vi "MSScript_Exe_Command.vi"(8 "error in (no error)":errorcluster, 9 "Expression index":i32, 11 "MSScript in":refnum<class "MSScript.lvclass">) -> (0 "Error out":errorcluster, 1 "Next expression index":i32, 3 "MSScript out":refnum<class "MSScript.lvclass">)   [LabVIEW 2018, in "MSScript.lvclass"]
uses:
  MSScript.lvclass
  MSScript.lvclass/MSScript.ctl
  MSScript_Error_(6008)UnknownCmd.vi
  MSScript_Error_(6007)CalcError.vi
  MSScript_Error_(6006)ParamErr.vi
  MSScript_Error_(6010)CommentLost.vi
  MSScript_Error_(6000)VariableNoFound.vi
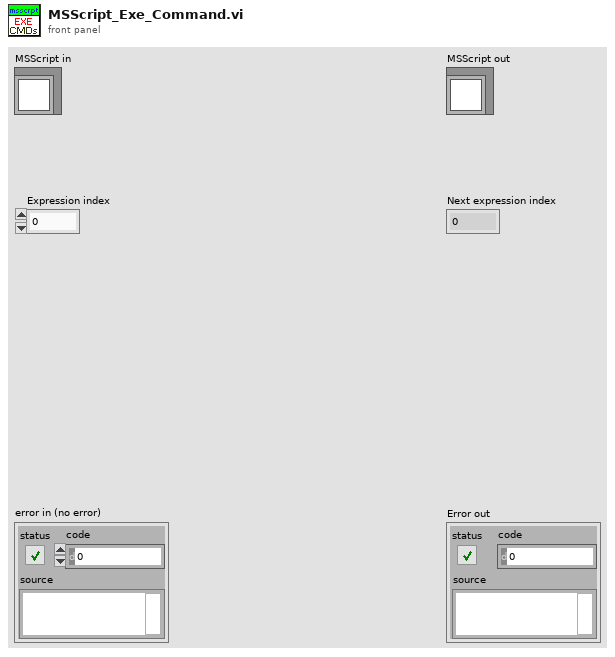
[diagram p1: front panel]
types:
  T1 = cluster{"Type":string, "NAME":cluster{"STR":string, "Start":i32}, "PARAMs":cluster{"STR":string, "Start":i32}[]}[]
  T2 = cluster{"Type":string, "NAME":cluster{"STR":string, "Start":i32}, "PARAMs":cluster{"STR":string, "Start":i32}[]}
  T3 = enum16{"Scalar", "ScalarArray", "Var", "VarArray", "Error"}
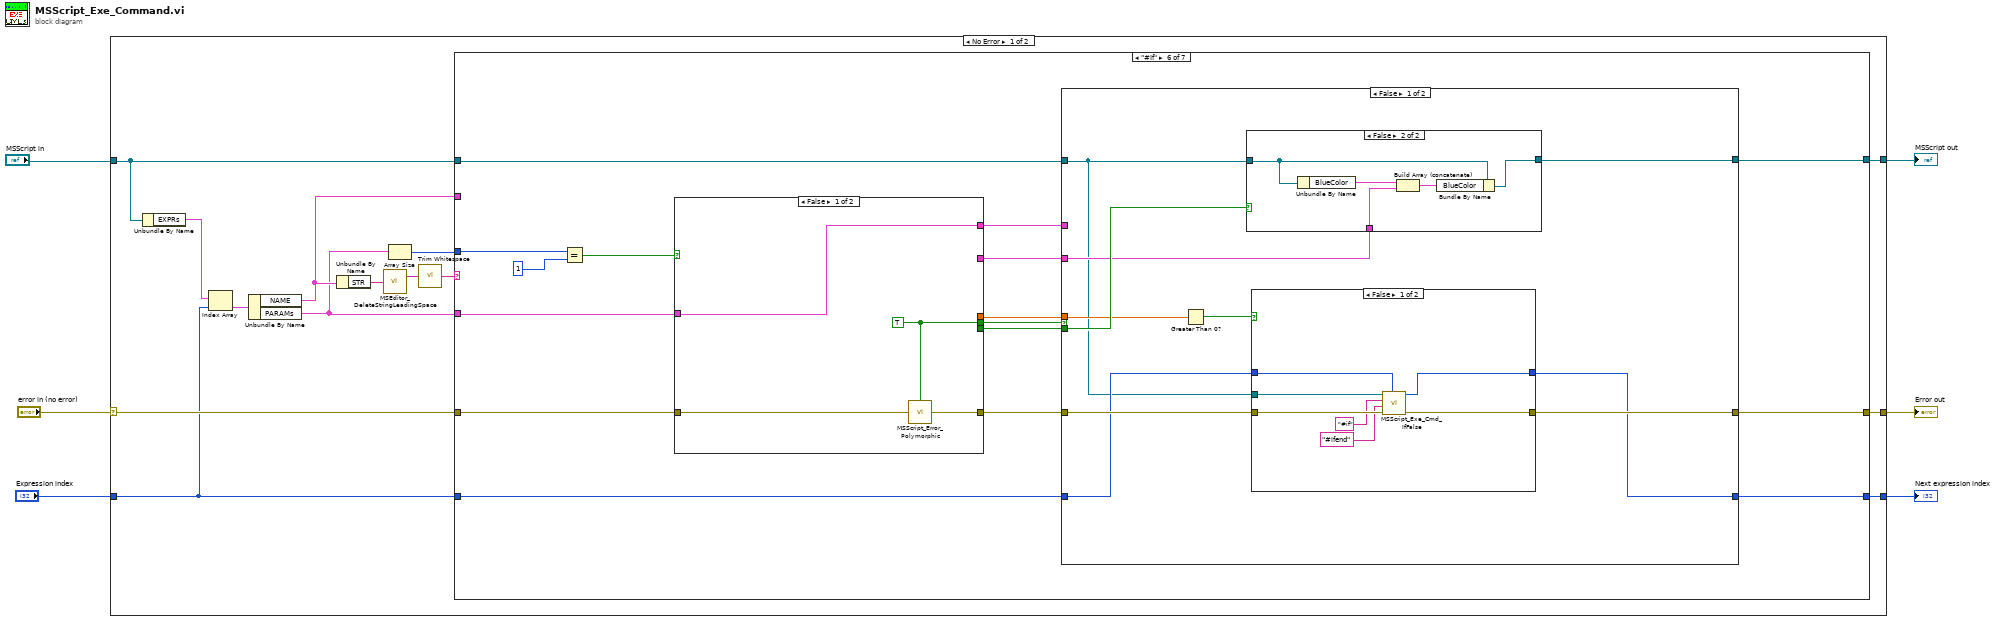
[diagram p0: block diagram]
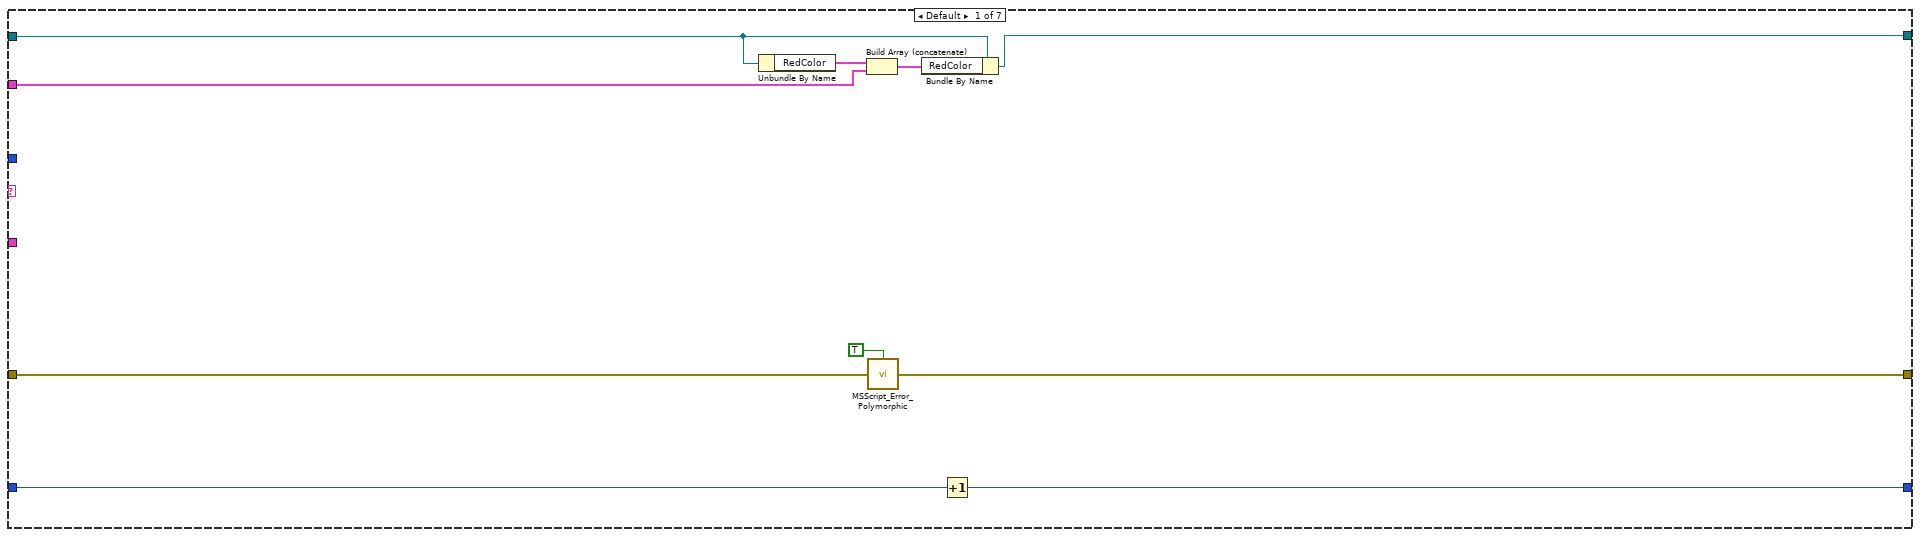
[diagram p2: hidden frame]
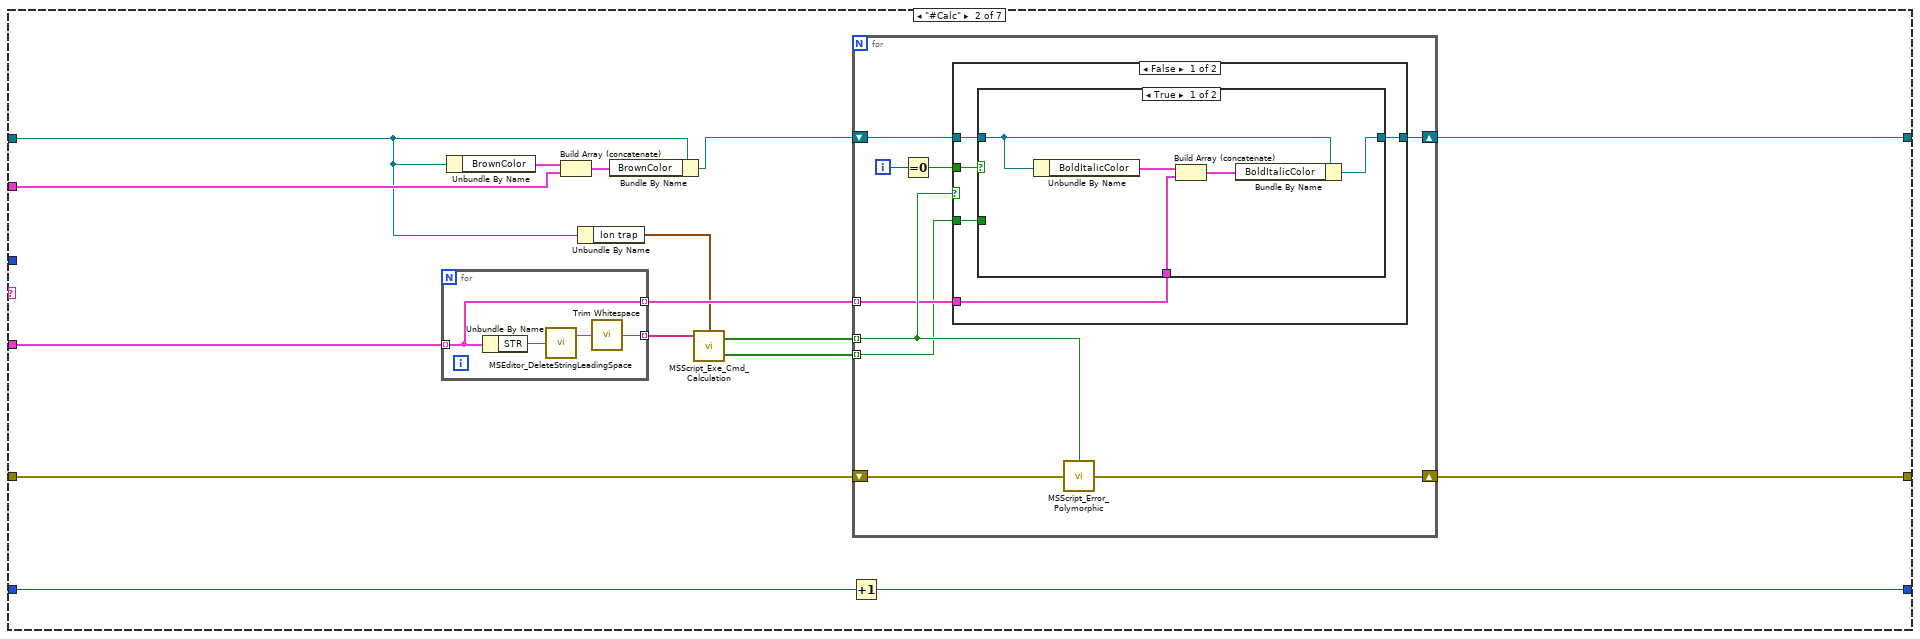
[diagram p3: hidden frame]
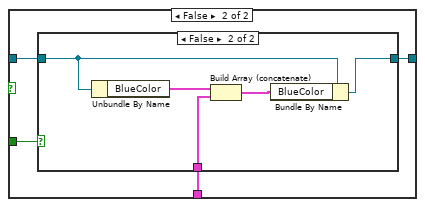
[diagram p4: hidden frame]
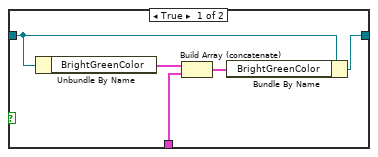
[diagram p5: hidden frame]
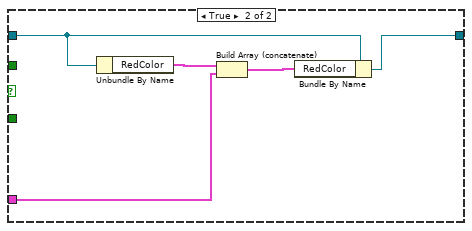
[diagram p6: hidden frame]
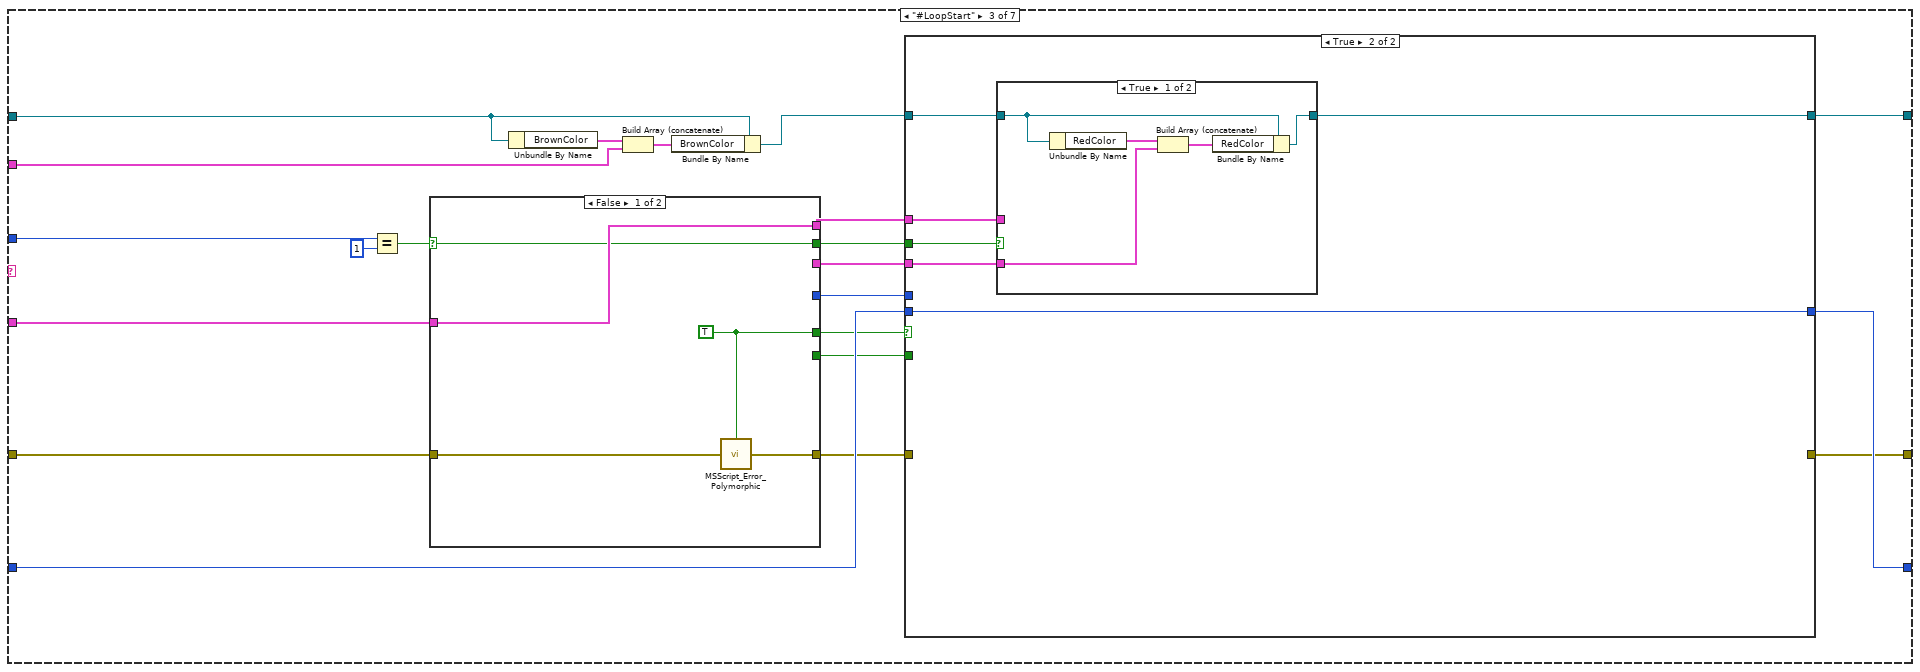
[diagram p7: hidden frame]
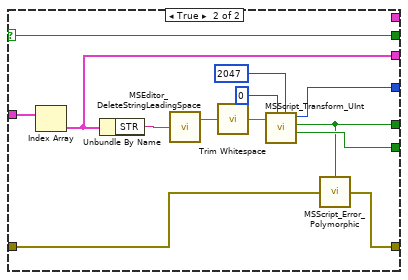
[diagram p8: hidden frame]
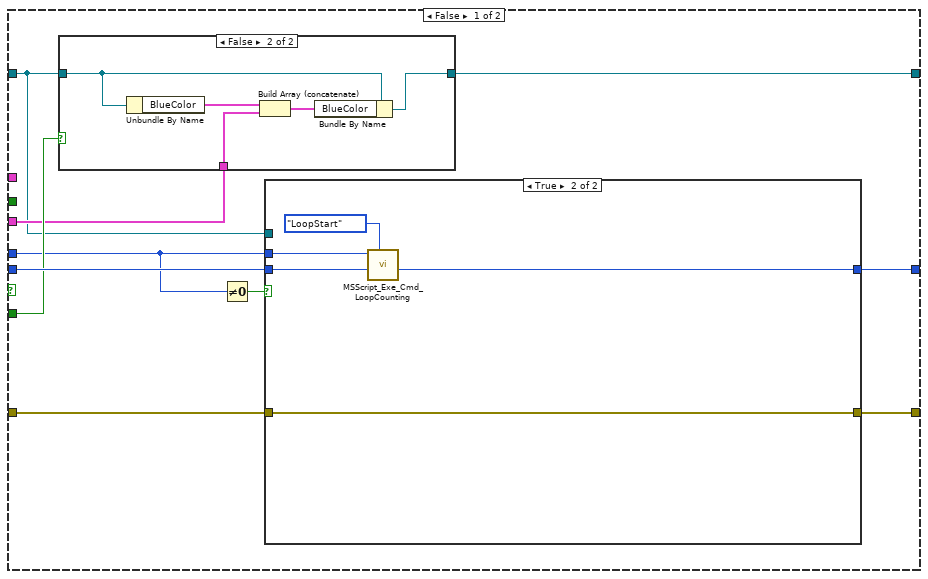
[diagram p9: hidden frame]
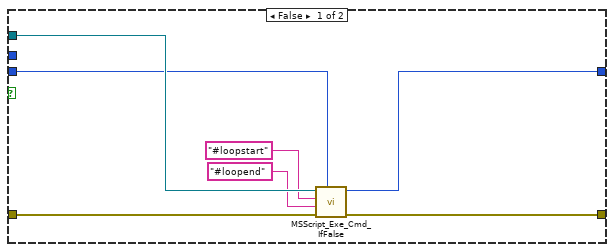
[diagram p10: hidden frame]
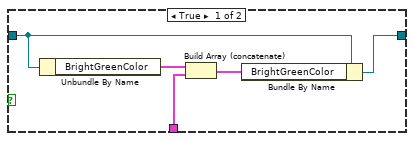
[diagram p11: hidden frame]
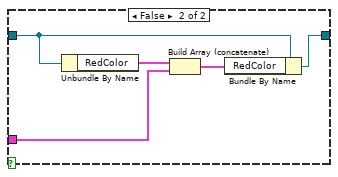
[diagram p12: hidden frame]
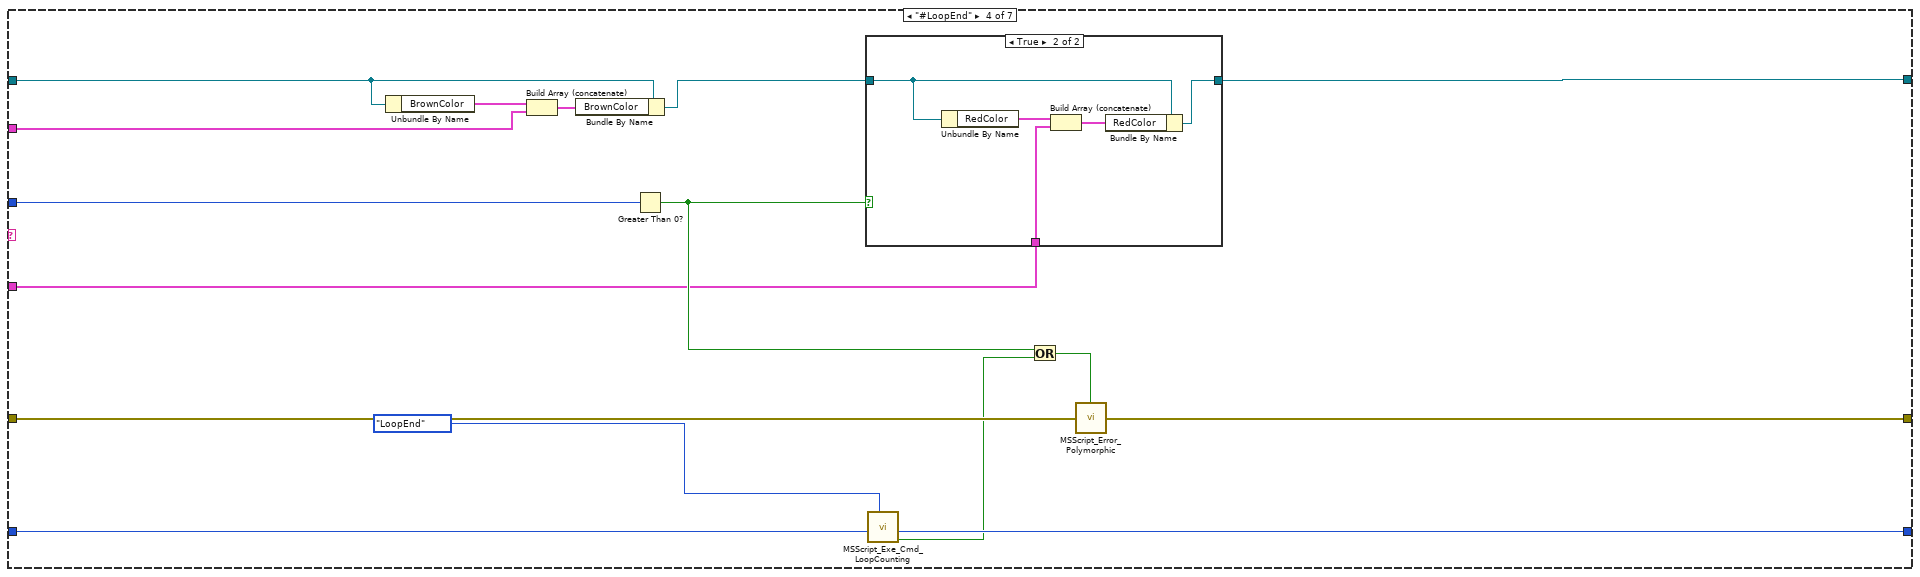
[diagram p13: hidden frame]
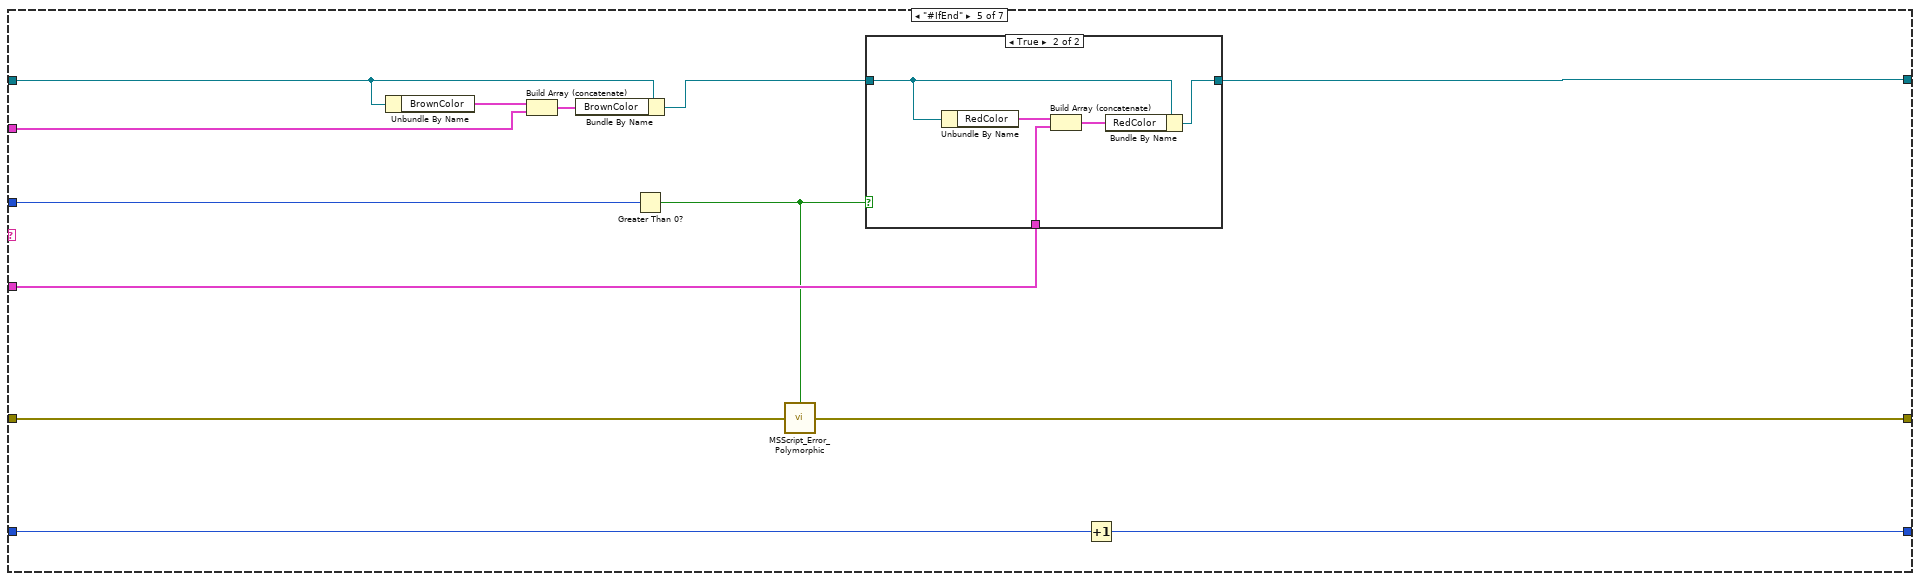
[diagram p15: hidden frame]
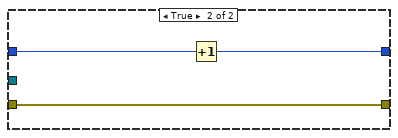
[diagram p17: hidden frame]
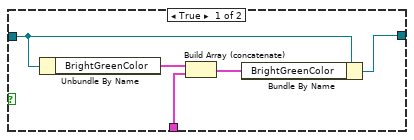
[diagram p18: hidden frame]
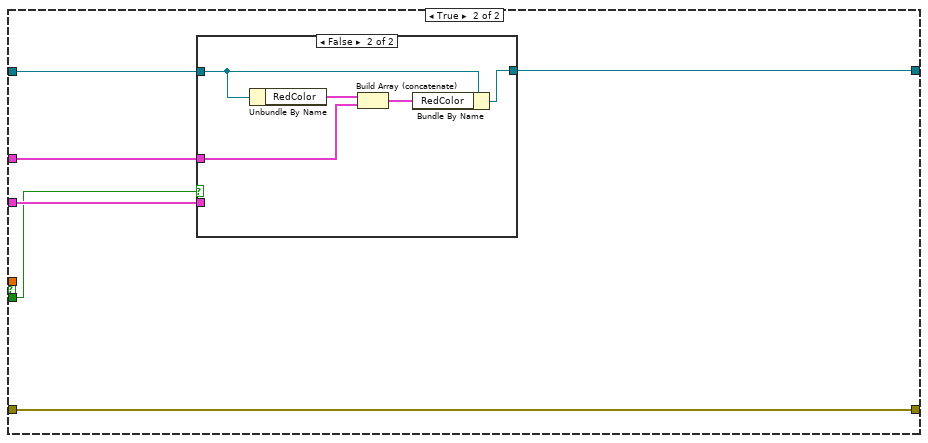
[diagram p19: hidden frame]
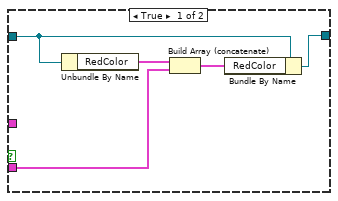
[diagram p20: hidden frame]
diagram:
  n1 = case shown="No Error" "error in (no error)" {
    selector: "error in (no error)" -> [w17 w388]
    tunnel: [w20 w386] -> w6
    tunnel: "MSScript in" -> [w7 w385]
    tunnel: "Expression index" -> [w8 w387]
    tunnel: [w16 w388] -> w2
    tunnel: [w12 w385] -> w1
    frame No Error {
      n2 = Unbundle By Name(w7) -> ("EXPRs"=w19:T1)
      n3 = Index Array(array=w19, index=w8) -> (element=w18:T2)
      n4 = Unbundle By Name(w18) -> ("NAME"=w11:cluster{"STR":string, "Start":i32}, "PARAMs"=w10:cluster{"STR":string, "Start":i32}[])
      n5 = Unbundle By Name(w11) -> ("STR"=w15:string)
      n6 = call "MSEditor_DeleteStringLeadingSpace.vi"("string in"=w15) -> ("string after leading space"=w14:string)  [unwired: 1 out]
      n7 = Array Size(array=w10) -> (size(s)=w9:i32)
      n8 = call <vilib>:"Trim Whitespace.vi"("string"=w14) -> ("trimmed string"=w13:string)  [unwired: 1 in]
      n9 = case shown="\"#If\"" w13 {
        tunnel: w10 -> [_ w44 w109 w176 w201 w228 w312]
        tunnel: w8 -> [w29 w45 w108 w190 w200 w218 w316]
        tunnel: [w30 w46 w107 w189 w199 w217 w317] -> w20
        tunnel: w17 -> [w28 w43 w106 w188 w210 w232 w305]
        tunnel: [w27 w42 w89 w187 w209 w221 w296] -> w16
        tunnel: w11 -> [w23 w36 w104 w185 w207 _ w315]
        tunnel: w7 -> [w22 w32 w105 w186 w208 w224 w314]
        tunnel: [w21 w34 w103 w177 w202 w220 w313] -> w12
        tunnel: w9 -> [_ _ w102 w184 w206 w230 w311]
        frame Default {
          n10 = Unbundle By Name(w22) -> ("RedColor"=w25:cluster{"STR":string, "Start":i32}[])
          n11 = Build Array (concatenate)(w25, w23) -> (w24:cluster{"STR":string, "Start":i32}[])
          n12 = call-poly "MSScript_Error_Polymorphic.vi"("error in (no error)"=w28, "ErrBoolean"=TRUE) -> ("error out"=w27:errorcluster)
          n13 = Bundle By Name(cluster=w22, "RedColor"=w24) -> (w21:refnum<class "MSScript.lvclass">)
          n14 = Increment(x=w29) -> (x+1=w30:i32)
        }
        frame "#Calc" {
          n15 = for {
            tunnel: w44 -> [w85] mode=indexing
            tunnel: [w86] -> w41 mode=indexing
            tunnel: [w85] -> w39 mode=indexing
            n16 = Unbundle By Name(w85) -> ("STR"=w87:string)
            n17 = call "MSEditor_DeleteStringLeadingSpace.vi"("string in"=w87) -> ("string after leading space"=w88:string)  [unwired: 1 out]
            n18 = call <vilib>:"Trim Whitespace.vi"("string"=w88) -> ("trimmed string"=w86:string)  [unwired: 1 in]
          }
          n19 = Unbundle By Name(w32) -> ("BrownColor"=w38:cluster{"STR":string, "Start":i32}[])
          n20 = Build Array (concatenate)(w38, w36) -> (w37:cluster{"STR":string, "Start":i32}[])
          n21 = Unbundle By Name(w32) -> ("Ion trap"=w31:cluster{"R0":ext, "Z0":ext})
          n22 = Bundle By Name(cluster=w32, "BrownColor"=w37) -> (w35:refnum<class "MSScript.lvclass">)
          n23 = call "MSScript_Exe_Cmd_Calculation.vi"("Ion trap"=w31, "ValueArray"=w41) -> ("Is a variable?"=w33:bool[], "ErrorBooleanArray"=w40:bool[])  [unwired: 2 in]
          n24 = Increment(x=w45) -> (x+1=w46:i32)
          n25 = for {
            tunnel: w40 -> [w51] mode=indexing
            shift-right: [w54] -> w42
            shift-left: w43 -> [w55]
            tunnel: w39 -> [w50] mode=indexing
            tunnel: w33 -> [w49] mode=indexing
            shift-right: [w53] -> w34
            shift-left: w35 -> [w52]
            i -> [w48]
            n26 = Equal To 0?(x=w48) -> (x = 0?=w47:bool)
            n27 = case shown="False" w51 {
              tunnel: [w59 w83] -> w53
              tunnel: w52 -> [w60 w84]
              tunnel: w50 -> [w58 w81]
              tunnel: w49 -> [w57 _]
              tunnel: w47 -> [w56 _]
              frame False {
                n28 = case shown="True" w56 {
                  tunnel: w60 -> [w63 w69]
                  tunnel: [w62 w68] -> w59
                  tunnel: w58 -> [w61 w67]
                  tunnel: w57 -> [_ w66]
                  frame True {
                    n29 = Unbundle By Name(w63) -> ("BoldItalicColor"=w65:cluster{"STR":string, "Start":i32}[])
                    n30 = Build Array (concatenate)(w65, w61) -> (w64:cluster{"STR":string, "Start":i32}[])
                    n31 = Bundle By Name(cluster=w63, "BoldItalicColor"=w64) -> (w62:refnum<class "MSScript.lvclass">)
                  }
                  frame False {
                    n32 = case shown="False" w66 {
                      tunnel: w69 -> [w74 w79]
                      tunnel: [w73 w78] -> w68
                      tunnel: w67 -> [w71 w76]
                      frame True {
                        n33 = Unbundle By Name(w74) -> ("BrightGreenColor"=w72:cluster{"STR":string, "Start":i32}[])
                        n34 = Build Array (concatenate)(w72, w71) -> (w70:cluster{"STR":string, "Start":i32}[])
                        n35 = Bundle By Name(cluster=w74, "BrightGreenColor"=w70) -> (w73:refnum<class "MSScript.lvclass">)
                      }
                      frame False {
                        n36 = Unbundle By Name(w79) -> ("BlueColor"=w77:cluster{"STR":string, "Start":i32}[])
                        n37 = Build Array (concatenate)(w77, w76) -> (w75:cluster{"STR":string, "Start":i32}[])
                        n38 = Bundle By Name(cluster=w79, "BlueColor"=w75) -> (w78:refnum<class "MSScript.lvclass">)
                      }
                    }
                  }
                }
              }
              frame True {
                n39 = Unbundle By Name(w84) -> ("RedColor"=w82:cluster{"STR":string, "Start":i32}[])
                n40 = Build Array (concatenate)(w82, w81) -> (w80:cluster{"STR":string, "Start":i32}[])
                n41 = Bundle By Name(cluster=w84, "RedColor"=w80) -> (w83:refnum<class "MSScript.lvclass">)
              }
            }
            n42 = call-poly "MSScript_Error_Polymorphic.vi"("error in (no error)"=w55, "ErrBoolean"=w51) -> ("error out"=w54:errorcluster)
          }
        }
        frame "#LoopStart" {
          n43 = Equal?(x=w102, y=1) -> (x = y?=w100:bool)
          n44 = case shown="False" w100 {
            selector: w100 -> [w113 w118]
            tunnel: w109 -> [w114 w127]
            tunnel: [_ w124] -> w99
            tunnel: [_ w120] -> w98
            tunnel: [w110 w115] -> w95
            tunnel: [_ w119] -> w93
            tunnel: [w114 _] -> w92
            tunnel: [w113 w118] -> w91
            tunnel: w106 -> [w112 w117]
            tunnel: [w111 w116] -> w90
            frame False {
              w110 = TRUE
              n45 = call-poly "MSScript_Error_Polymorphic.vi"("error in (no error)"=w112, "ErrBoolean"=w110) -> ("error out"=w111:errorcluster)
            }
            frame True {
              n46 = Index Array(array=w127) -> (element=w120:cluster{"STR":string, "Start":i32})  [unwired: 1 in]
              n47 = Unbundle By Name(w120) -> ("STR"=w122:string)
              n48 = call "MSEditor_DeleteStringLeadingSpace.vi"("string in"=w122) -> ("string after leading space"=w123:string)  [unwired: 1 out]
              n49 = call <vilib>:"Trim Whitespace.vi"("string"=w123) -> ("trimmed string"=w121:string)  [unwired: 1 in]
              n50 = call "MSScript_Transform_UInt.vi"("upper limit"=u64 2047, "lower limit"=u64 0, "string in"=w121) -> ("Is a variable ?"=w119:bool, "Value Error?"=w115:bool, "Value Output"=w124:u64)  [unwired: 6 in]
              n51 = call-poly "MSScript_Error_Polymorphic.vi"("error in (no error)"=w117, "ErrBoolean"=w115) -> ("error out"=w116:errorcluster)
            }
          }
          n52 = Unbundle By Name(w105) -> ("BrownColor"=w97:cluster{"STR":string, "Start":i32}[])
          n53 = Build Array (concatenate)(w97, w104) -> (w96:cluster{"STR":string, "Start":i32}[])
          n54 = Bundle By Name(cluster=w105, "BrownColor"=w96) -> (w94:refnum<class "MSScript.lvclass">)
          n55 = case shown="True" w95 {
            tunnel: w108 -> [w137 w165]
            tunnel: [w136 w165] -> w107
            tunnel: w99 -> [w132 _]
            tunnel: w98 -> [w133 w164]
            tunnel: [w135 w162] -> w103
            tunnel: w94 -> [w130 w163]
            tunnel: w93 -> [w134 _]
            tunnel: w92 -> [_ w161]
            tunnel: w91 -> [_ w160]
            tunnel: w90 -> [w129 _]
            tunnel: [w128 _] -> w89
            frame False {
              n56 = case shown="False" w134 {
                tunnel: w130 -> [w152 w157]
                tunnel: [w151 w156] -> w135
                tunnel: w133 -> [w150 w155]
                frame True {
                  n57 = Unbundle By Name(w152) -> ("BrightGreenColor"=w154:cluster{"STR":string, "Start":i32}[])
                  n58 = Build Array (concatenate)(w154, w150) -> (w153:cluster{"STR":string, "Start":i32}[])
                  n59 = Bundle By Name(cluster=w152, "BrightGreenColor"=w153) -> (w151:refnum<class "MSScript.lvclass">)
                }
                frame False {
                  n60 = Unbundle By Name(w157) -> ("BlueColor"=w159:cluster{"STR":string, "Start":i32}[])
                  n61 = Build Array (concatenate)(w159, w155) -> (w158:cluster{"STR":string, "Start":i32}[])
                  n62 = Bundle By Name(cluster=w157, "BlueColor"=w158) -> (w156:refnum<class "MSScript.lvclass">)
                }
              }
              n63 = Not Equal To 0?(x=w132) -> (x != 0?=w131:bool)
              n64 = case shown="True" w131 {
                tunnel: w137 -> [w139 w149]
                tunnel: [w141 w148] -> w136
                tunnel: w132 -> [_ w146]
                tunnel: w130 -> [w144 _]
                tunnel: w129 -> [w143 w145]
                tunnel: [w142 w145] -> w128
                frame False {
                  n65 = call "MSScript_Exe_Cmd_IfFalse.vi"("Index"=w139, "error in (no error)"=w143, "End"="#loopend" ("Start"), "Start"="#loopstart", "MSScript in"=w144) -> ("Error out"=w142:errorcluster, "Index of the next sentence"=w141:i32)  [unwired: 3 in]
                }
                frame True {
                  n66 = call "MSScript_Exe_Cmd_LoopCounting.vi"("Function"=enum16{"Init", "LoopStart", "LoopEnd"}."LoopStart", "Index"=w149, "Times"=w146) -> ("Index of the next sentence"=w148:i32)  [unwired: 7 in, 1 out]
                }
              }
            }
            frame True {
              n67 = case shown="True" w160 {
                tunnel: w164 -> [w168 _]
                tunnel: w163 -> [w167 w173]
                tunnel: [w166 w172] -> w162
                tunnel: w161 -> [_ w171]
                frame True {
                  n68 = Unbundle By Name(w167) -> ("RedColor"=w170:cluster{"STR":string, "Start":i32}[])
                  n69 = Build Array (concatenate)(w170, w168) -> (w169:cluster{"STR":string, "Start":i32}[])
                  n70 = Bundle By Name(cluster=w167, "RedColor"=w169) -> (w166:refnum<class "MSScript.lvclass">)
                }
                frame False {
                  n71 = Unbundle By Name(w173) -> ("RedColor"=w175:cluster{"STR":string, "Start":i32}[])
                  n72 = Build Array (concatenate)(w175, w171) -> (w174:cluster{"STR":string, "Start":i32}[])
                  n73 = Bundle By Name(cluster=w173, "RedColor"=w174) -> (w172:refnum<class "MSScript.lvclass">)
                }
              }
            }
          }
        }
        frame "#LoopEnd" {
          n74 = Unbundle By Name(w186) -> ("BrownColor"=w181:cluster{"STR":string, "Start":i32}[])
          n75 = Build Array (concatenate)(w181, w185) -> (w180:cluster{"STR":string, "Start":i32}[])
          n76 = Bundle By Name(cluster=w186, "BrownColor"=w180) -> (w178:refnum<class "MSScript.lvclass">)
          n77 = Greater Than 0?(x=w184) -> (x > 0?=w179:bool)
          n78 = case shown="True" w179 {
            tunnel: w178 -> [w192 w194]
            tunnel: [w192 w193] -> w177
            tunnel: w176 -> [_ w195]
            frame False {
            }
            frame True {
              n79 = Unbundle By Name(w194) -> ("RedColor"=w197:cluster{"STR":string, "Start":i32}[])
              n80 = Build Array (concatenate)(w197, w195) -> (w196:cluster{"STR":string, "Start":i32}[])
              n81 = Bundle By Name(cluster=w194, "RedColor"=w196) -> (w193:refnum<class "MSScript.lvclass">)
            }
          }
          n82 = call "MSScript_Exe_Cmd_LoopCounting.vi"("Function"=enum16{"Init", "LoopStart", "LoopEnd"}."LoopEnd", "Index"=w190) -> ("Error?"=w183:bool, "Index of the next sentence"=w189:i32)  [unwired: 8 in]
          n83 = Or(x=w179, y=w183) -> (x .or. y?=w182:bool)
          n84 = call-poly "MSScript_Error_Polymorphic.vi"("error in (no error)"=w188, "ErrBoolean"=w182) -> ("error out"=w187:errorcluster)
        }
        frame "#IfEnd" {
          n85 = Unbundle By Name(w208) -> ("BrownColor"=w205:cluster{"STR":string, "Start":i32}[])
          n86 = Build Array (concatenate)(w205, w207) -> (w204:cluster{"STR":string, "Start":i32}[])
          n87 = Bundle By Name(cluster=w208, "BrownColor"=w204) -> (w203:refnum<class "MSScript.lvclass">)
          n88 = Greater Than 0?(x=w206) -> (x > 0?=w198:bool)
          n89 = call-poly "MSScript_Error_Polymorphic.vi"("error in (no error)"=w210, "ErrBoolean"=w198) -> ("error out"=w209:errorcluster)
          n90 = case shown="True" w198 {
            tunnel: w203 -> [w211 w213]
            tunnel: [w211 w212] -> w202
            tunnel: w201 -> [_ w214]
            frame False {
            }
            frame True {
              n91 = Unbundle By Name(w213) -> ("RedColor"=w216:cluster{"STR":string, "Start":i32}[])
              n92 = Build Array (concatenate)(w216, w214) -> (w215:cluster{"STR":string, "Start":i32}[])
              n93 = Bundle By Name(cluster=w213, "RedColor"=w215) -> (w212:refnum<class "MSScript.lvclass">)
            }
          }
          n94 = Increment(x=w200) -> (x+1=w199:i32)
        }
        frame "#If" {
          n95 = Equal?(x=w230, y=1) -> (x = y?=w229:bool)
          n96 = case shown="False" w229 {
            tunnel: w228 -> [w282 w294]
            tunnel: [_ w287] -> w219
            tunnel: [_ w291] -> w226
            tunnel: [w279 w286] -> w227
            tunnel: [w282 _] -> w225
            tunnel: w232 -> [w281 w290]
            tunnel: [w280 w289] -> w223
            tunnel: [_ w283] -> w222
            frame False {
              w279 = TRUE
              n97 = call-poly "MSScript_Error_Polymorphic.vi"("error in (no error)"=w281, "ErrBoolean"=w279) -> ("error out"=w280:errorcluster)
            }
            frame True {
              n98 = Index Array(array=w294) -> (element=w291:cluster{"STR":string, "Start":i32})  [unwired: 1 in]
              n99 = Unbundle By Name(w291) -> ("STR"=w292:string)
              n100 = call "MSEditor_DeleteStringLeadingSpace.vi"("string in"=w292) -> ("string after leading space"=w293:string)  [unwired: 1 out]
              n101 = call <vilib>:"Trim Whitespace.vi"("string"=w293) -> ("trimmed string"=w288:string)  [unwired: 1 in]
              n102 = call "MSScript_Transform_Extended.vi"("upper limit (Inf)"=ext inf, "lower limit (-Inf)"=ext -inf, "Check_Str"=w288) -> ("Is a variable ?"=w283:bool, "Value Error?"=w286:bool, "Value Output"=w287:ext)  [unwired: 6 in]
              n103 = call-poly "MSScript_Error_Polymorphic.vi"("error in (no error)"=w290, "ErrBoolean"=w286) -> ("error out"=w289:errorcluster)
            }
          }
          n104 = case shown="False" w227 {
            tunnel: w226 -> [w240 w268]
            tunnel: [w242 w266] -> w220
            tunnel: w224 -> [w233 w267]
            tunnel: w222 -> [w241 w263]
            tunnel: w225 -> [_ w265]
            tunnel: w223 -> [w239 w264]
            tunnel: [w238 w264] -> w221
            tunnel: w219 -> [w237 _]
            tunnel: w218 -> [w235 _]
            tunnel: [w234 _] -> w217
            frame False {
              n105 = Greater Than 0?(x=w237) -> (x > 0?=w236:bool)
              n106 = case shown="False" w241 {
                tunnel: w233 -> [w255 w260]
                tunnel: [w254 w259] -> w242
                tunnel: w240 -> [w253 w258]
                frame True {
                  n107 = Unbundle By Name(w255) -> ("BrightGreenColor"=w257:cluster{"STR":string, "Start":i32}[])
                  n108 = Build Array (concatenate)(w257, w253) -> (w256:cluster{"STR":string, "Start":i32}[])
                  n109 = Bundle By Name(cluster=w255, "BrightGreenColor"=w256) -> (w254:refnum<class "MSScript.lvclass">)
                }
                frame False {
                  n110 = Unbundle By Name(w260) -> ("BlueColor"=w262:cluster{"STR":string, "Start":i32}[])
                  n111 = Build Array (concatenate)(w262, w258) -> (w261:cluster{"STR":string, "Start":i32}[])
                  n112 = Bundle By Name(cluster=w260, "BlueColor"=w261) -> (w259:refnum<class "MSScript.lvclass">)
                }
              }
              n113 = case shown="False" w236 {
                tunnel: w235 -> [w249 w251]
                tunnel: [w248 w250] -> w234
                tunnel: w239 -> [w247 w252]
                tunnel: [w246 w252] -> w238
                tunnel: w233 -> [w243 _]
                frame False {
                  n114 = call "MSScript_Exe_Cmd_IfFalse.vi"("Index"=w249, "error in (no error)"=w247, "End"="#ifend", "Start"="#if", "MSScript in"=w243) -> ("Error out"=w246:errorcluster, "Index of the next sentence"=w248:i32)  [unwired: 3 in]
                }
                frame True {
                  n115 = Increment(x=w251) -> (x+1=w250:i32)
                }
              }
            }
            frame True {
              n116 = case shown="False" w263 {
                tunnel: w268 -> [w271 _]
                tunnel: w267 -> [w270 w276]
                tunnel: [w269 w275] -> w266
                tunnel: w265 -> [_ w274]
                frame True {
                  n117 = Unbundle By Name(w270) -> ("RedColor"=w273:cluster{"STR":string, "Start":i32}[])
                  n118 = Build Array (concatenate)(w273, w271) -> (w272:cluster{"STR":string, "Start":i32}[])
                  n119 = Bundle By Name(cluster=w270, "RedColor"=w272) -> (w269:refnum<class "MSScript.lvclass">)
                }
                frame False {
                  n120 = Unbundle By Name(w276) -> ("RedColor"=w278:cluster{"STR":string, "Start":i32}[])
                  n121 = Build Array (concatenate)(w278, w274) -> (w277:cluster{"STR":string, "Start":i32}[])
                  n122 = Bundle By Name(cluster=w276, "RedColor"=w277) -> (w275:refnum<class "MSScript.lvclass">)
                }
              }
            }
          }
        }
        frame "#Show" {
          n123 = Less Or Equal?(x=w311, y=2) -> (x <= y?=w306:bool)
          n124 = case shown="True" w306 {
            tunnel: w312 -> [w348 w359]
            tunnel: [w348 w359] -> w307
            tunnel: [_ w356] -> w298
            tunnel: [_ w370] -> w299
            tunnel: [w346 w360] -> w303
            tunnel: [w352 w368] -> w302
            tunnel: w305 -> [w350 w367]
            tunnel: [_ w358] -> w304
            tunnel: [_ w357] -> w297
            tunnel: [_ w355] -> w295
            frame False {
              n125 = Array Size(array=w348) -> (size(s)=w347:i32)
              n126 = call-poly "MSScript_Error_Polymorphic.vi"("error in (no error)"=w350, "ErrBoolean"=TRUE ("Error?")) -> ("error out"=w352:errorcluster)
              n127 = Initialize Array(TRUE, w347) -> (w346:bool[])
            }
            frame True {
              n128 = Index Array(array=w359, index #1=0 ("index"), index #2=1 ("index")) -> (element #1=w369:cluster{"STR":string, "Start":i32}, element #2=w364:cluster{"STR":string, "Start":i32})
              n129 = Unbundle By Name(w364) -> ("STR"=w363:string)
              n130 = Unbundle By Name(w369) -> ("STR"=w354:string)
              n131 = call "_PC_Pub_Conv_ColorHexNum.vi"("HexStringIn"=w363) -> ("ErrorBool"=w361:bool, "HexNumOut"=w357:u32)  [unwired: 1 in]
              n132 = call "MSScript_SubVI_VarTypeIden.vi"("Var in"=w354) -> ("Type"=w353:T3)
              n133 = case shown="\"VarArray\"" w353 {
                tunnel: [_ w374 w380] -> w370
                tunnel: [TRUE ("Error?") w378 w381] -> w362
                tunnel: [TRUE ("Is a variable ?") w377 w382] -> w358
                tunnel: w354 -> [w373 w376 w384]
                tunnel: [w373 w376 w383] -> w356
                tunnel: [_ _ w379] -> w355
                frame "Error", Default {
                }
                frame "Var" {
                  n134 = call "MSScript_SubVI_ScalarVariableAccess.vi"("VarName"=w376) -> ("Value Error?"=w378:bool, "OutputValue"=w375:ext, "Is a variable ?"=w377:bool)  [unwired: 6 in]
                  n135 = Build Array(w375) -> (w374:ext[])
                }
                frame "VarArray" {
                  n136 = call "MSScript_SubVI_GetShowArray.vi"("VarString in"=w384) -> ("ArrayVariable out"=w380:ext[], "Index"=w379:i32[], "ShowName"=w383:string, "Is a variable ?"=w382:bool, "Value Error?"=w381:bool)  [unwired: 6 in]
                }
              }
              n137 = Build Array(w362, w361) -> (w360:bool[])
              n138 = call-poly "MSScript_Error_Polymorphic.vi"("error in (no error)"=w367, "ErrBoolean"=w362) -> ("error out"=w368:errorcluster)
            }
          }
          n139 = Unbundle By Name(w314) -> ("BrownColor"=w309:cluster{"STR":string, "Start":i32}[])
          n140 = Build Array (concatenate)(w309, w315) -> (w308:cluster{"STR":string, "Start":i32}[])
          n141 = Bundle By Name(cluster=w314, "BrownColor"=w308) -> (w301:refnum<class "MSScript.lvclass">)
          n142 = for {
            tunnel: w307 -> [w321] mode=indexing
            tunnel: w304 -> [w318]
            shift-right: [w323] -> w313
            shift-left: w301 -> [w322]
            tunnel: w303 -> [w320] mode=indexing
            i -> [w319]
            n143 = case shown="False" w320 {
              tunnel: [w330 w342] -> w323
              tunnel: w322 -> [w325 w343]
              tunnel: w321 -> [w329 w341]
              tunnel: w319 -> [w327 _]
              tunnel: w318 -> [w324 _]
              frame False {
                n144 = Equal To 0?(x=w327) -> (x = 0?=w326:bool)
                n145 = And(x=w326, y=w324) -> (x .and. y?=w328:bool)
                n146 = case shown="True" w328 {
                  tunnel: w325 -> [w333 w338]
                  tunnel: [w332 w337] -> w330
                  tunnel: w329 -> [w331 w336]
                  frame False {
                    n147 = Unbundle By Name(w333) -> ("BlueColor"=w335:cluster{"STR":string, "Start":i32}[])
                    n148 = Build Array (concatenate)(w335, w331) -> (w334:cluster{"STR":string, "Start":i32}[])
                    n149 = Bundle By Name(cluster=w333, "BlueColor"=w334) -> (w332:refnum<class "MSScript.lvclass">)
                  }
                  frame True {
                    n150 = Unbundle By Name(w338) -> ("BrightGreenColor"=w340:cluster{"STR":string, "Start":i32}[])
                    n151 = Build Array (concatenate)(w340, w336) -> (w339:cluster{"STR":string, "Start":i32}[])
                    n152 = Bundle By Name(cluster=w338, "BrightGreenColor"=w339) -> (w337:refnum<class "MSScript.lvclass">)
                  }
                }
              }
              frame True {
                n153 = Unbundle By Name(w343) -> ("RedColor"=w345:cluster{"STR":string, "Start":i32}[])
                n154 = Build Array (concatenate)(w345, w341) -> (w344:cluster{"STR":string, "Start":i32}[])
                n155 = Bundle By Name(cluster=w343, "RedColor"=w344) -> (w342:refnum<class "MSScript.lvclass">)
              }
            }
          }
          n156 = Increment(x=w316) -> (x+1=w317:i32)
          n157 = Unbundle By Name(w301) -> ("Listbox Ref"=w300:refnum<vi>)
          n158 = call "MSScript_SubVI_EditorShowTo.vi"("Listbox Ref"=w300, "Variable In"=w299, "Variable Index"=w295, "Variable Name"=w298, "error in (no error)"=w302, "String Color"=w297) -> ("error out"=w296:errorcluster)  [unwired: 9 in]
        }
      }
    }
    frame Error {
      (unwired) TRUE ("Executes the next sentence")
      n159 = Increment(x=w387) -> (x+1=w386:i32)
    }
  }
  "Next expression index" <- w6
  "Error out" <- w2
  "MSScript out" <- w1
